vi "Toggle Defer.vi"(6 "Defer":bool, 8 "error in":errorcluster, 11 "Report Viewer in":refnum<class "Report Viewer.lvclass">) -> (0 "error out":errorcluster, 3 "Report Viewer out":refnum<class "Report Viewer.lvclass">)   [LabVIEW 2019, in "Report Viewer.lvlib" / "Report Viewer.lvclass"]
uses:
  Library/Report Viewer.lvclass
  Library/Report Viewer.lvclass/Report Viewer.ctl
  Accessors/GUI/Read VI Refnum.vi
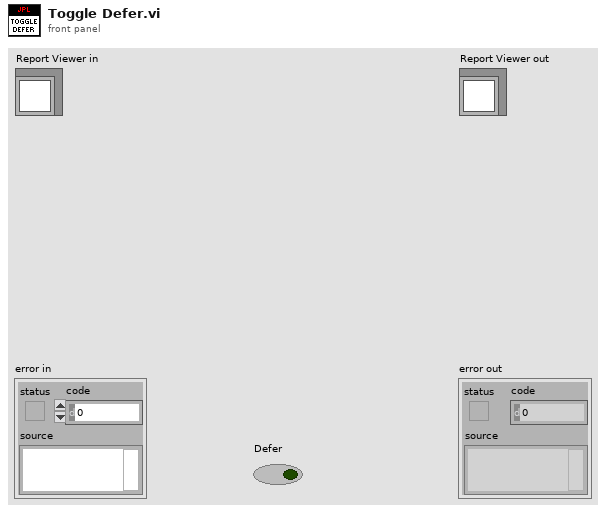
[diagram p1: front panel]
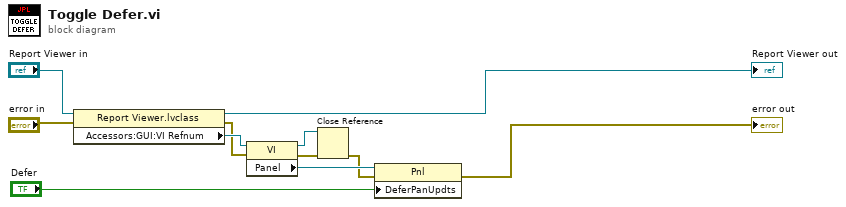
[diagram p0: block diagram]
diagram:
  n1 = property class="Report Viewer.lvclass"(reference="Report Viewer in", error in="error in") -> (reference out=→"Report Viewer out":refnum<class "Report Viewer.lvclass">, error out=w1:errorcluster, "Accessors:GUI:VI Refnum"=w2:refnum<vi>)
  n2 = property class="VI"(reference=w2, error in=w1) -> (reference out=w11:refnum<vi>, error out=w10:errorcluster, "Panel"=w9:refnum<vi>)
  n3 = Close Reference(reference=w11, error in (no error)=w10) -> (error out=w7:errorcluster)
  n4 = property class="Pnl"(reference=w9, error in=w7, "DeferPanUpdts"="Defer") -> (error out=→"error out":errorcluster)  [unwired: 1 out]
